vi "getRowElements.vi"(8 "error in (no error)":errorcluster, 11 "Outcome in":refnum<class "Outcome.lvclass">) -> (0 "error out":errorcluster, 2 "Row Interface":string[](array[string]), 3 "Outcome out":refnum<class "Outcome.lvclass">)   [LabVIEW 2020]
uses:
  Outcome.lvclass
  Outcome.lvclass/Outcome.ctl
  Goal/Goal.lvclass
  C:/GitRepos/Filthy-Lucre-Budgetizer/source/support/classes/Expense Summary/Outcome.lvclass
  C:/GitRepos/Filthy-Lucre-Budgetizer/source/support/classes/RowDisplayable/RowRepresentable.lvclass
  C:/GitRepos/Filthy-Lucre-Budgetizer/source/support/classes/UserEditableAmount/UserEditableAmount.lvclass
  C:/GitRepos/Filthy-Lucre-Budgetizer/source/support/classes/Goal/Goal.lvclass
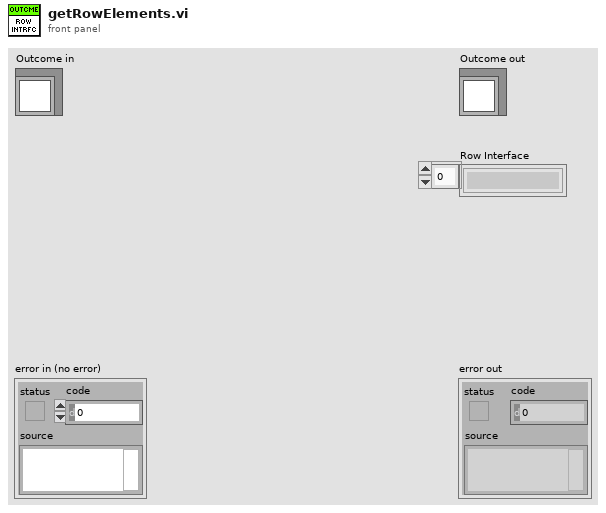
[diagram p1: front panel]
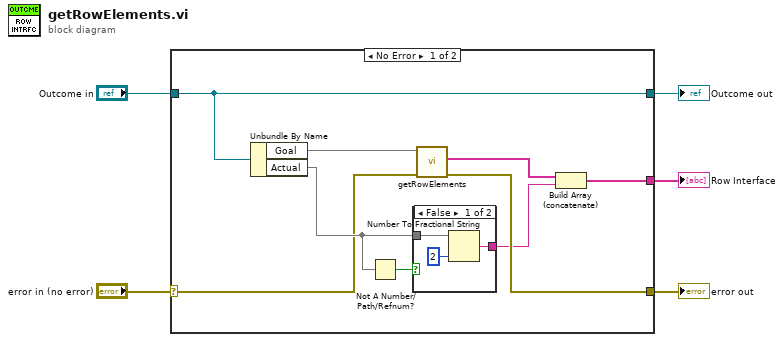
[diagram p0: block diagram]
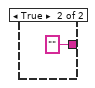
[diagram p2: hidden frame]
diagram:
  n1 = case shown="No Error" "error in (no error)" {
    selector: "error in (no error)" -> [w6 w20]
    tunnel: [w11 w20] -> w4
    tunnel: [w14 w19] -> w2
    tunnel: "Outcome in" -> [w14 w19]
    tunnel: [w8 _] -> w1
    frame No Error {
      n2 = Unbundle By Name(w14) -> ("Goal"=w7, "Actual"=w12)
      n3 = Not A Number/Path/Refnum?(number/path/refnum=w12) -> (NaN/Path/Refnum?=w13:bool)
      n4 = case shown="False" w13 {
        tunnel: [w16 ""] -> w9
        tunnel: w12 -> [w15 _]
        frame False {
          n5 = Number To Fractional String(number=w15, precision (6)=i16 2) -> (F-format string=w16:string)  [unwired: 2 in]
        }
        frame True {
        }
      }
      n6 = call-dynamic "getRowElements.vi"("error in (no error)"=w6, "Goal in"=w7) -> ("error out"=w11:errorcluster, "Row Interface"=w10:string[])  [unwired: 7 in, 1 out]
      n7 = Build Array (concatenate)(w10, w9) -> (w8:string[])
    }
    frame Error {
    }
  }
  "error out" <- w4
  "Outcome out" <- w2
  "Row Interface" <- w1
